vi "programa 11.vi"() -> ()   [LabVIEW 2012]
uses:
  Control del programa 11.ctl
panel:
  out "Array":dbl[][](array[numeric])
  # "Ingresar numeros enteros entre 1-200, luego en la ultima linea del arreglo\nreservarla para obtener el numero mayor de cada una de las columnas."
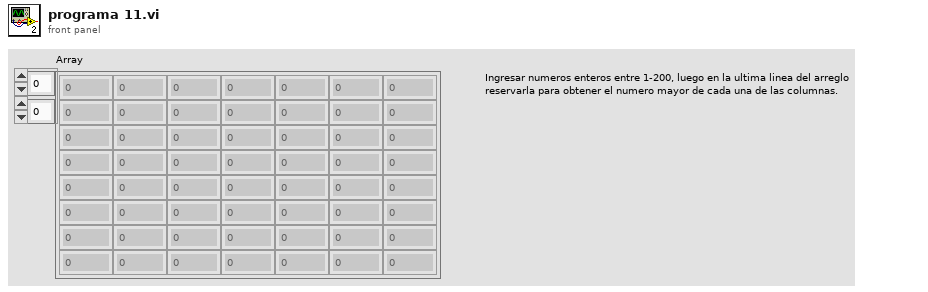
[diagram p1: front panel]
types:
  T1 = typedef "Control del programa 11.ctl" = enum16{"Inicializar", "Rellenar", "Mayor de cada columna", "Finalizar"}
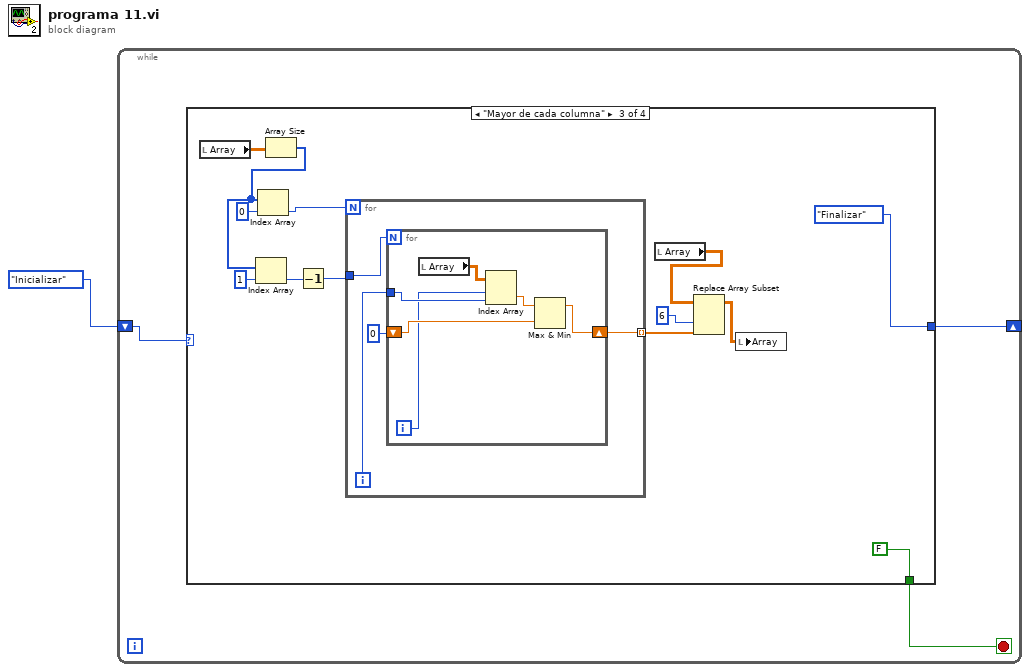
[diagram p0: block diagram]
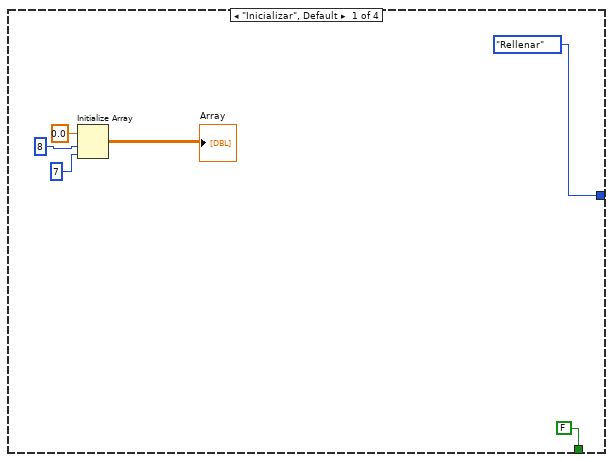
[diagram p2: hidden frame]
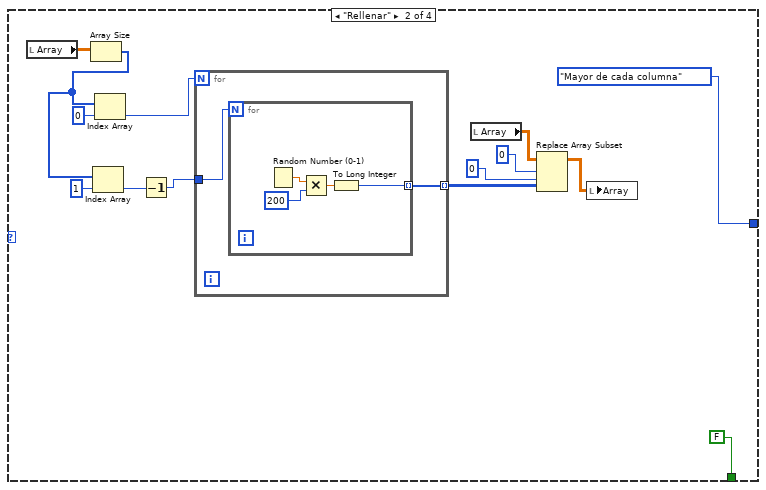
[diagram p3: hidden frame]
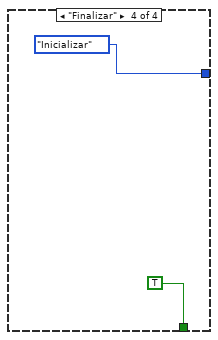
[diagram p4: hidden frame]
diagram:
  n1 = while {
    shift-right: [w3] -> _
    shift-left: Control_del_programa_11."Inicializar" -> [w4]
    stop <- w2 stop-if-true
    n2 = case shown="\"Mayor de cada columna\"" w4 {
      tunnel: [Control_del_programa_11."Rellenar" Control_del_programa_11."Mayor de cada columna" Control_del_programa_11."Finalizar" Control_del_programa_11."Inicializar"] -> w3
      tunnel: [FALSE FALSE FALSE TRUE] -> w2
      frame "Inicializar", Default {
        n3 = Initialize Array "Initialize Array"(0.0 ("element"), 8, 7) -> (→"Array":dbl[][])
      }
      frame "Rellenar" {
        n4 = local read "Array"() -> (w24:dbl[][])
        n5 = Array Size(array=w24) -> (size(s)=w23:i32[])
        n6 = Index Array "Index Array"(array=w23, index=1) -> (element=w13:i32)
        n7 = Index Array "Index Array"(array=w23, index=0) -> (element=w11:i32)
        n8 = Decrement(x=w13) -> (x-1=w12:i32)
        n9 = for {
          N: w11 -> [_]
          tunnel: w12 -> [w26]
          tunnel: [w25] -> w18 mode=indexing
          n10 = for {
            N: w26 -> [_]
            tunnel: [w27] -> w25 mode=indexing
            n11 = Random Number (0-1)() -> (number: 0 to 1=w30:dbl)
            n12 = Multiply(x=w30, y=200) -> (x*y=w28:dbl)
            n13 = To Long Integer(number=w28) -> (32bit integer=w27:i32)
          }
        }
        n14 = local read "Array"() -> (w20:dbl[][])
        n15 = Replace Array Subset "Replace Array Subset"(array=w20, new element=w18, index (row)=0, index (col)=0) -> (w19:dbl[][])
        n16 = local write "Array"(w19) -> ()
      }
      frame "Mayor de cada columna" {
        n17 = local read "Array"() -> (w43:dbl[][])
        n18 = Array Size(array=w43) -> (size(s)=w42:i32[])
        n19 = Index Array "Index Array"(array=w42, index=1) -> (element=w33:i32)
        n20 = Index Array "Index Array"(array=w42, index=0) -> (element=w31:i32)
        n21 = Decrement(x=w33) -> (x-1=w32:i32)
        n22 = for {
          N: w31 -> [_]
          tunnel: w32 -> [w47]
          tunnel: [w44] -> w38 mode=indexing
          i -> [w46]
          n23 = for {
            N: w47 -> [_]
            tunnel: w46 -> [w49]
            shift-right: [w50] -> w44
            shift-left: 0 -> [w51]
            i -> [w48]
            n24 = local read "Array"() -> (w53:dbl[][])
            n25 = Index Array "Index Array"(array=w53, index (row)=w48, index (col)=w49) -> (element=w52:dbl)
            n26 = Max & Min(x=w52, y=w51) -> (max(x,y)=w50:dbl)  [unwired: 1 out]
          }
        }
        n27 = local read "Array"() -> (w39:dbl[][])
        n28 = Replace Array Subset "Replace Array Subset"(array=w39, new element=w38, index (col)=6 ("disabled index (col)")) -> (w37:dbl[][])  [unwired: 1 in]
        n29 = local write "Array"(w37) -> ()
      }
      frame "Finalizar" {
      }
    }
  }
